vi "UDP - Sender.vi"(8 "error in (no error)":errorcluster, 11 "destination address":string="255.255.255.255") -> (0 "error out":errorcluster, 2 "log file path":path, 3 "Results":string[][](array[string]))   [LabVIEW 2019]
doc: "The UDP protocol differs from TCP in that there is no error-checking with the packets of information that are sent, and thus no guarantee whatsoever that an intended recipient will actually receive a given piece of data.\n\nUDP does offer the ability to \"broadcast\" data across a network--simply specify an IP Address of all ones (255.255.255.255) to attempt to broadcast information network-wide. Keep in mind that routers and other network hardware will generally refuse to forward the broadcast beyond certain points, so the extent of the broadcast will in practice be limited."
panel:
  in  "ports to check":u16[](array[numeric])=[44515, 44525]
  out "log file name":string
  out "Current test":cluster{string, "error out":errorcluster}
  out "current port":u16
  in  "Start Test":bool
  out "current value":dbl
  # "Overview: Sends UDP data to the destination addresses. Set destination address to the server address or to 255.255.255.255 to send to the entire network.\n\nInstructions:\n1. Run the VI and click Start Test\n2. Open Simple UDP - Receiver.vi and follow the instructions on its front panel.\n3. Click Stop to stop the VI."
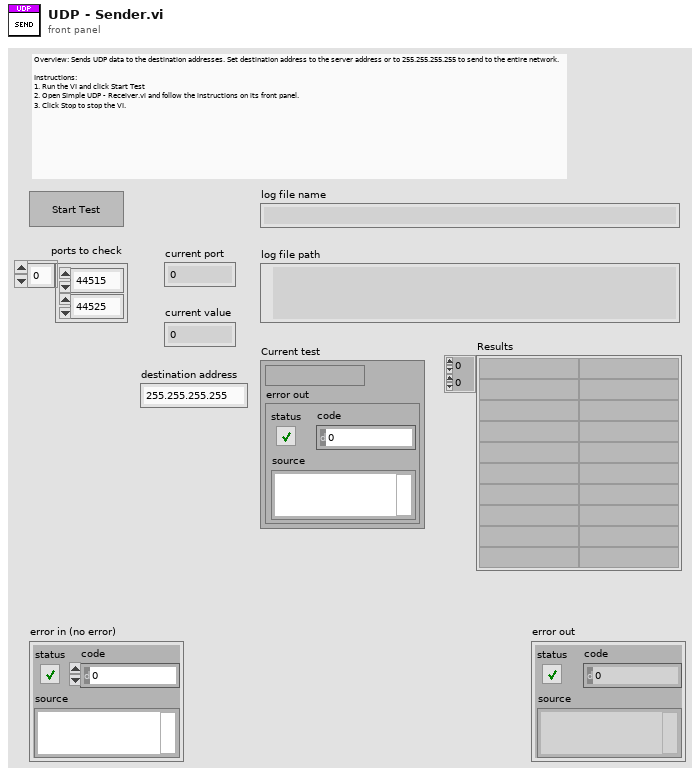
[diagram p1: front panel]
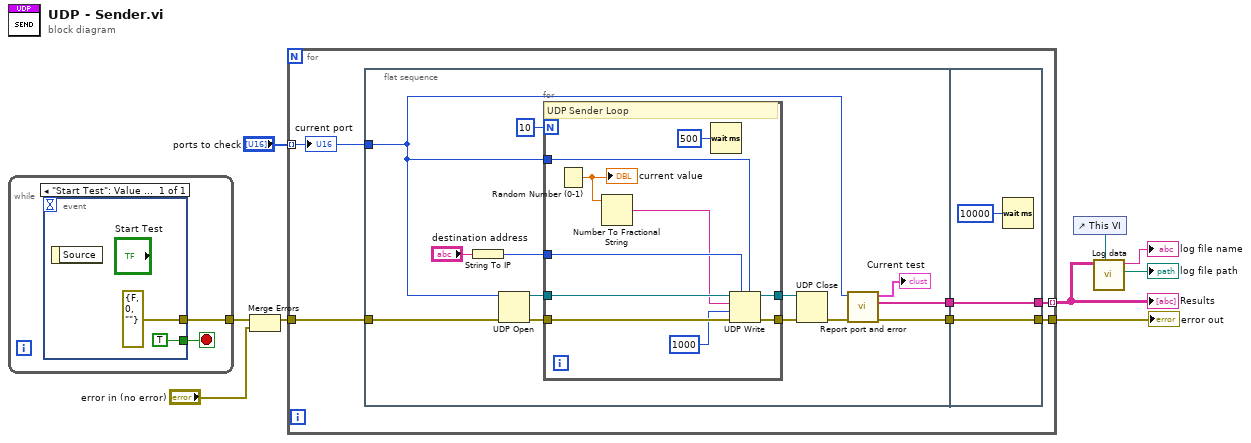
[diagram p0: block diagram]
diagram:
  n1 = while {
    tunnel: [w11] -> w4
    stop <- w10 stop-if-true
    n2 = event shown="[0] \"Start Test\": Value Change" {
      selector: _ -> [_]
      dyn-events: _ -> [_]
      timeout: _ -> [_]
      tunnel: [errorcluster {"status"=FALSE, "code"=0, "source"=""} ("error constant")] -> w11
      tunnel: [TRUE] -> w10
      event "Start Test": Value Change {
        n3 = event-data() -> ()  [unwired: 1 in, 1 out]
      }
    }
  }
  n4 = Merge Errors(w4, "error in (no error)") -> (w3:errorcluster)
  n5 = for {
    tunnel: "ports to check" -> [w17] mode=indexing
    tunnel: w3 -> [w16]
    tunnel: [w18] -> w5 mode=indexing
    tunnel: [w14] -> w1
    n6 = flat-sequence {
      tunnel: w17 -> [w21]
      tunnel: [w23] -> w19
      tunnel: w16 -> [w22]
      tunnel: [w20] -> w15
      tunnel: [w45] -> w18
      tunnel: w19 -> [w45]
      tunnel: [w43] -> w14
      tunnel: w15 -> [w43]
      frame #0 {
        n7 = String To IP(1:"destination address") -> (0:w29:u32)
        n8 = UDP Open(8:w22, 11:w21) -> (port=w28:refnum<k16>, 0:w27:errorcluster)  [unwired: 3 in, 1 out]
        n9 = for {
          N: 10 -> [_]
          tunnel: [w34] -> w31
          tunnel: w28 -> [w42]
          tunnel: w27 -> [w41]
          tunnel: [w40] -> w32
          tunnel: w29 -> [w39]
          tunnel: w21 -> [w36]
          # "UDP Sender Loop"
          n10 = Random Number (0-1)() -> (number: 0 to 1=w35:dbl)
          "current value" <- w35
          n11 = Number To Fractional String(number=w35) -> (F-format string=w37:string)  [unwired: 3 in]
          n12 = Wait (ms)(milliseconds to wait=u32 500) -> ()  [unwired: 1 out]
          n13 = UDP Write(address=w39, port or service name=w36, connection ID=w42, data in=w37, 8:w41, 9:1000 ("timeout ms (25000)")) -> (error out=w34:errorcluster, 3:w40:refnum<k16>)
        }
        n14 = UDP Close(connection ID=w32, 8:w31) -> (error out=w25:errorcluster)  [unwired: 1 out]
        n15 = call "Report port and error.vi"("error in (no error)"=w25, "port"=w21) -> ("error out"=w20:errorcluster, "Array"=w23:string[], "output cluster"=→"Current test":cluster{string, "error out":errorcluster})  [unwired: 7 in]
      }
      frame #1 {
        n16 = Wait (ms)(milliseconds to wait=u32 10000) -> ()  [unwired: 1 out]
      }
    }
    "current port" <- w17
  }
  "Results" <- w5
  "error out" <- w1
  n17 = control-ref of="This VI"() -> (w6:refnum<vi>)
  n18 = call "Log data.vi"("reference"=w6, "Data"=w5) -> ("log file path"=→"log file path":path, "log file name"=→"log file name":string)  [unwired: 7 in, 1 out]
